vi "Manual CAN Send Cammand.vi"() -> ()   [LabVIEW 2015]
panel:
  in  "stop":bool
  out "number":u32[](array[numeric])
  out "appended array":string[](array[string])
  out "all rows":string[][](array[string])
  in  "CAN  Send Cammand":bool
  in  "Responce Cammand":string
  in  "Cammand Test":u16(ring) items=["Send req seed send key to test sample", "Send Diag command to sample", "Buzzer ON", "Buzzer OFF", "End Activation command to test sample", "Send req seed send key to master", "Send Diag command to master", "Send req seed send key to test sample", "Send Diag command to Test sample", "Dial Illumination ON for master", "Pointer Illumination ON for master", "LCD Illumination ON for master", "Dial Illumination ON for Test Sample", "Pointer Illumination ON for Test Sample", "LCD Illumination ON for Test Sample", "LCD All Seg ON to master", "LCD All Seg ON to test sample", "LCD All segment OFF to master", "LCD All segment OFF to test sample", "End Activation command to master", "End Activation command to test sample", "All telltale ON command to master", "All telltale ON command to test sample", "All telltlae OFF command to master", "All telltlae OFF command to test sample", "End Activation command for Master", "End Activation command for Test", "Move Speedo to 0 km/hr to master", "Move Speedo to 0 km/hr to Test sample", "Move speedo to 20 km/hr to master", "Move speedo to 20 km/hr to test sample", "Move speedo to 40 km/hr to master", "Move speedo to 40 km/hr to test sample", "Move speedo to 60 km/hr to master", "Move speedo to 60 km/hr to test sample", "Move Speedo to 80 km/hr to master", "Move Speedo to 80 km/hr to test sample", "Move speedo to 100 km/hr to master", "Move speedo to 100 km/hr to test sample", "Move Speedo to 120 to master", "Move Speedo to 120 to test sample", "Move speedo to 140 km/hr to master", "Move speedo to 140 km/hr to test sample", "Move speedo to 160 km/hr to master", "Move speedo to 160 km/hr to test sample", "Move Speedo to 180 to master", "Move Speedo to 180 to test sample", "End Activation for Testing Sample", "Send req seed send key to test sample", "Send Diag command to Test sample", "CLEAR DTC LID 95", "CLEAR DTC LID 96", "CLEAR DTC LID 97", "CLEAR DTC LID 98", "CLEAR DTC LID 99", "CLEAR DTC LID 9A", "CLEAR DTC LID 9B", "CLEAR DTC LID 9C", "CLEAR DTC LID 9D", "CLEAR DTC LID 9E", "CLEAR DTC LID 9F", "CLEAR DTC LID A0", "CLEAR DTC LID A1", "CLEAR DTC LID A2", "CLEAR DTC LID A3", "CLEAR DTC LID A4", "CLEAR DTC LID A5", "CLEAR DTC LID A6", "CLEAR DTC LID A7", "CLEAR DTC LID A8", "CLEAR DTC LID A9", "CLEAR DTC LID AA", "READ DTC LID 95", "Read Request", "End Activation command to Master sample", "End Activation command to test sample"]
  out "Cammand":string
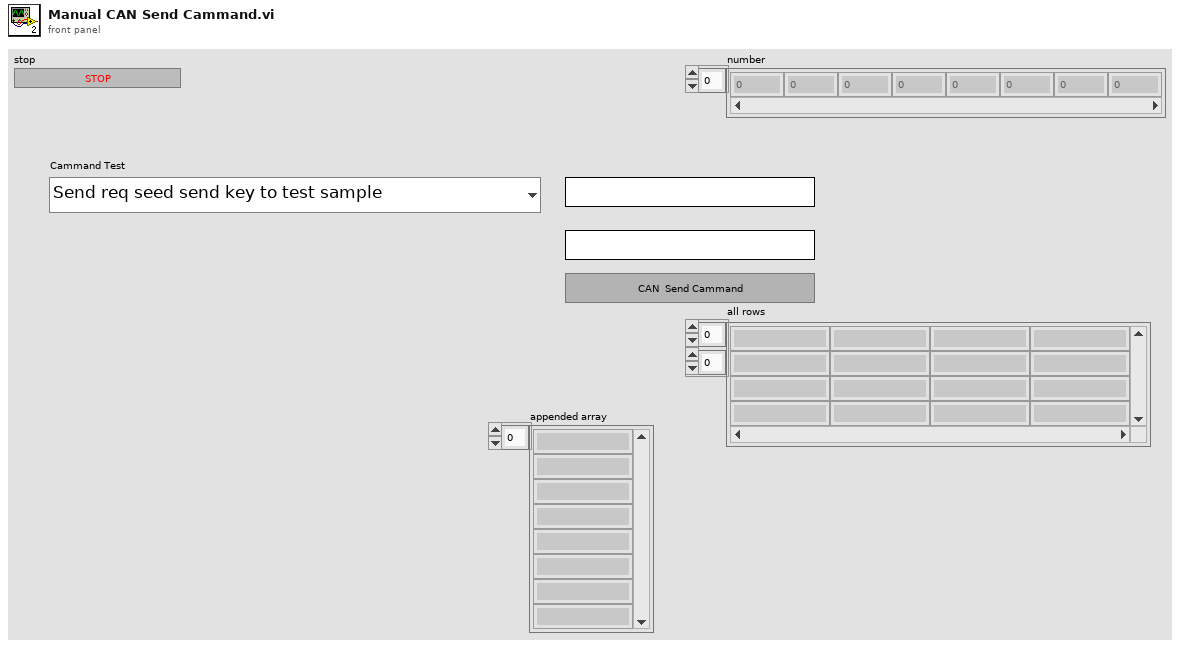
[diagram p1: front panel]
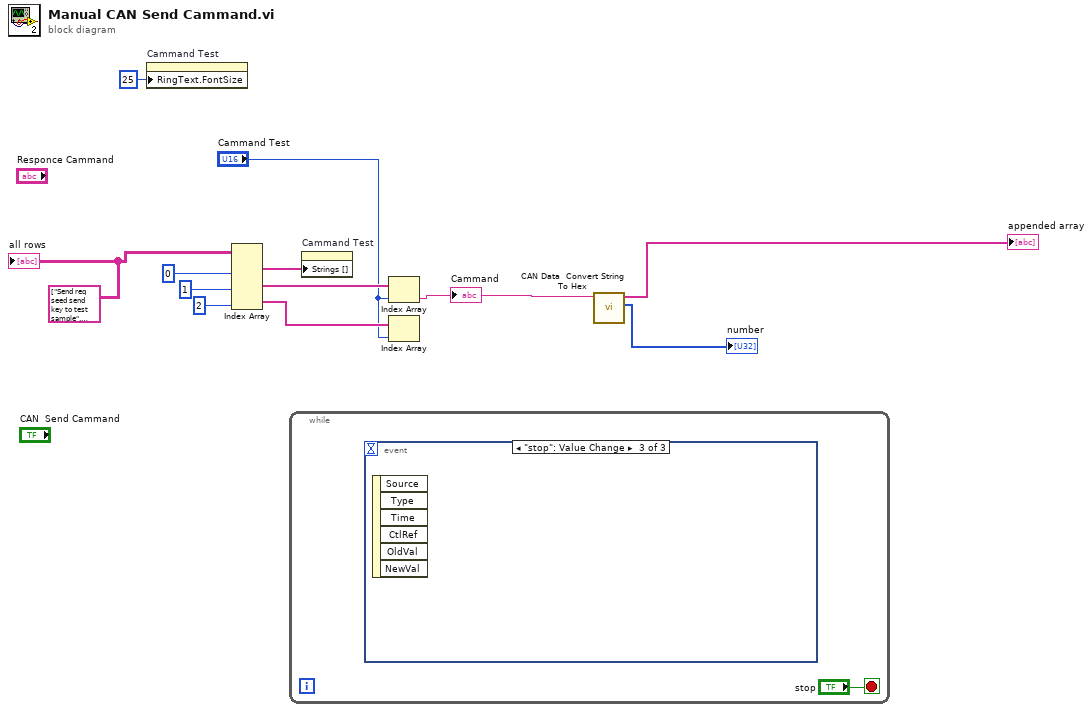
[diagram p0: block diagram]
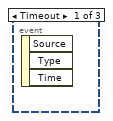
[diagram p2: hidden frame]
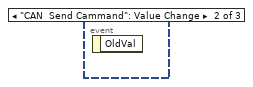
[diagram p3: hidden frame]
diagram:
  w1 = string[][] [["Send req seed send key to test sample", "0227FB0000000000", "0667FB", "0627FC", "0367FC34", "1", "0227FC", "0", "CAN0", "0", ""], ["Send Diag command to sample", "0210FA", "0250FA", "", "0", "0", "", "0", "CAN0", "0", ""], ["Buzzer ON", "0730130780800A00", "03701307", "", "", "0", "2", "0", "CAN0", "0", ""], ["Buzzer OFF", "0730130780800000", "03701307", "", "", "0", "", "0", "CAN0", "", ""], ["End Activation command to test sample", "0120", "0160", "", "", "0", "", "0", "CAN0", "0", ""], ["Send req seed send key to master", "0227FB0000000000", "0667FB", "0627FC", "0367FC34", "1", "24", "0", "CAN1", "0", ""], ["Send Diag command to master", "0210FA", "0250FA", "", "0", "0", "24", "0", "CAN1", "0", ""], ["Send req seed send key to test sample", "0227FB0000000000", "0667FB", "0627FC", "0367FC34", "1", "3", "0", "CAN0", "0", ""], ["Send Diag command to Test sample", "0210FA", "0250FA", "", "0", "0", "3", "0", "CAN0", "0", ""], ["Dial Illumination ON for master", "0631840100FFFF00", "027184", "", "", "0", "24", "0", "CAN1", "0", ""], ["Pointer Illumination ON for master", "0631840101FFFF00", "027184", "", "", "0", "24", "0", "CAN1", "0", ""], ["LCD Illumination ON for master", "0631840102FFFF00", "027160", "", "", "0", "24", "0", "CAN1", "0", ""], ["Dial Illumination ON for Test Sample", "0631840100FFFF00", "027184", "", "", "0", "4", "0", "CAN0", "0", ""], ["Pointer Illumination ON for Test Sample", "0631840101FFFF00", "027184", "", "", "0", "4", "0", "CAN0", "0", ""], ["LCD Illumination ON for Test Sample", "0631840102FFFF00", "027160", "", "", "0", "4", "0", "CAN0", "0", ""], ["LCD All Seg ON to master", "0431602100000000", "027160", "", "", "0", "24", "0", "CAN1", "0", ""], ["LCD All Seg ON to test sample", "0431602100000000", "027160", "", "", "0", "4", "0", "CAN0", "0", ""], ["LCD All segment OFF to master", "0431604100000000", "027160", "56", "0", "0", "24", "0", "CAN1", "0", ""], ["LCD All segment OFF to test sample", "0431604100000000", "027160", "56", "0", "0", "5", "0", "CAN0", "0", ""], ["End Activation command to master", "0120", "0160", "", "", "0", "24", "0", "CAN1", "0", ""], ["End Activation command to test sample", "0120", "0160", "", "", "0", "", "0", "CAN0", "0", ""], ["All telltale ON command to master", "0431342100", "027134", "", "", "0", "24", "1", "CAN1", "0", ""], ["All telltale ON command to test sample", "0431342100", "027134", "", "", "0", "6", "1", "CAN0", "0", ""], ["All telltlae OFF command to master", "0431344100", "027134", "", "", "0", "24", "1", "CAN1", "0", ""], ["All telltlae OFF command to test sample", "0431344100", "027134", "", "", "0", "7", "1", "CAN0", "0", ""], ["End Activation command for Master", "0120", "", "", "", "0", "24", "0", "CAN1", "0", ""], ["End Activation command for Test", "0120", "", "", "", "0", "8", "0", "CAN0", "0", ""], ["Move Speedo to 0 km/hr to master", "0000000000000000", "", "", "", "0", "24", "1", "CAN1", "788", ""], ["Move Speedo to 0 km/hr to Test sample", "0000000000000000", "", "", "", "0", "9", "1", "CAN0", "788", ""], ["Move speedo to 20 km/hr to master", "000A000000000000", "", "", "", "0", "24", "1", "CAN1", "788", ""], ["Move speedo to 20 km/hr to test sample", "000A000000000000", "", "", "", "0", "10", "1", "CAN0", "788", ""], ["Move speedo to 40 km/hr to master", "0014000000000000", "", "", "", "0", "24", "1", "CAN1", "788", ""], ["Move speedo to 40 km/hr to test sample", "0014000000000000", "", "", "", "0", "11", "1", "CAN0", "788", ""], ["Move speedo to 60 km/hr to master", "001E000000000000", "", "", "", "0", "24", "1", "CAN1", "788", ""], ["Move speedo to 60 km/hr to test sample", "001E000000000000", "", "", "", "0", "12", "1", "CAN0", "788", ""], ["Move Speedo to 80 km/hr to master", "0028000000000000", "", "", "", "0", "24", "1", "CAN1", "788", ""], ["Move Speedo to 80 km/hr to test sample", "0028000000000000", "", "", "", "0", "13", "1", "CAN0", "788", ""], ["Move speedo to 100 km/hr to master", "0032000000000000", "", "", "", "0", "24", "1", "CAN1", "788", ""], ["Move speedo to 100 km/hr to test sample", "0032000000000000", "", "", "", "0", "14", "1", "CAN0", "788", ""], ["Move Speedo to 120 to master", "003C000000000000", "", "", "", "0", "24", "1", "CAN1", "788", ""], ["Move Speedo to 120 to test sample", "003C000000000000", "", "", "", "0", "15", "1", "CAN0", "788", ""], ["Move speedo to 140 km/hr to master", "0046000000000000", "", "", "", "0", "24", "1", "CAN1", "788", ""], ["Move speedo to 140 km/hr to test sample", "0046000000000000", "", "", "", "0", "16", "1", "CAN0", "788", ""], ["Move speedo to 160 km/hr to master", "0050000000000000", "", "", "", "0", "24", "1", "CAN1", "788", ""], ["Move speedo to 160 km/hr to test sample", "0050000000000000", "", "", "", "0", "17", "1", "CAN0", "788", ""], ["Move Speedo to 180 to master", "005A000000000000", "", "", "", "0", "24", "1", "CAN1", "788", ""], ["Move Speedo to 180 to test sample", "005A000000000000", "", "", "", "0", "18", "1", "CAN0", "788", ""], ["End Activation for Testing Sample", "0120", "0160", "", "", "0", "", "0", "CAN0", "628", ""], ["Send req seed send key to test sample", "0227FB0000000000", "0667FB", "0627FC", "0367FC34", "1", "3", "0", "CAN0", "0", ""], ["Send Diag command to Test sample", "0210FA0000000000", "0250FA", "", "0", "0", "3", "0", "CAN0", "0", ""], ["CLEAR DTC LID 95", "0314FF000", "027161", "", "", "0", "22", "0", "CAN0", "0", ""], ["CLEAR DTC LID 96", "053161819600", "027161", "", "", "0", "", "0", "CAN0", "", ""], ["CLEAR DTC LID 97", "053161819700", "027161", "", "", "0", "", "0", "CAN0", "", ""], ["CLEAR DTC LID 98", "053161819800", "027161", "", "", "0", "", "0", "CAN0", "", ""], ["CLEAR DTC LID 99", "053161819900", "027161", "", "", "0", "", "0", "CAN0", "", ""], ["CLEAR DTC LID 9A", "053161819A00", "027161", "", "", "0", "", "0", "CAN0", "", ""], ["CLEAR DTC LID 9B", "053161819B00", "027161", "", "", "0", "", "0", "CAN0", "", ""], ["CLEAR DTC LID 9C", "053161819C00", "027161", "", "", "0", "", "0", "CAN0", "", ""], ["CLEAR DTC LID 9D", "053161819D00", "027161", "", "", "0", "", "0", "CAN0", "", ""], ["CLEAR DTC LID 9E", "053161819E00", "027161", "", "", "0", "", "0", "CAN0", "", ""], ["CLEAR DTC LID 9F", "053161819F00", "027161", "", "", "0", "", "0", "CAN0", "", ""], ["CLEAR DTC LID A0", "05316181A000", "027161", "", "", "0", "", "0", "CAN0", "", ""], ["CLEAR DTC LID A1", "05316181A100", "027161", "", "", "0", "", "0", "CAN0", "", ""], ["CLEAR DTC LID A2", "05316181A200", "027161", "", "", "0", "", "0", "CAN0", "", ""], ["CLEAR DTC LID A3", "05316181A300", "027161", "", "", "0", "", "0", "CAN0", "", ""], ["CLEAR DTC LID A4", "05316181A400", "027161", "", "", "0", "", "0", "CAN0", "", ""], ["CLEAR DTC LID A5", "05316181A500", "027161", "", "", "0", "", "0", "CAN0", "", ""], ["CLEAR DTC LID A6", "05316181A600", "027161", "", "", "0", "", "0", "CAN0", "", ""], ["CLEAR DTC LID A7", "05316181A700", "027161", "", "", "0", "", "0", "CAN0", "", ""], ["CLEAR DTC LID A8", "05316181A800", "027161", "", "", "0", "", "0", "CAN0", "", ""], ["CLEAR DTC LID A9", "05316181A900", "027161", "", "", "0", "", "0", "CAN0", "", ""], ["CLEAR DTC LID AA", "05316181AA00", "027161", "", "", "0", "", "0", "CAN0", "", ""], ["READ DTC LID 95", "0431610195000000", "02716100", "", "", "0", "", "0", "CAN0", "", ""], ["Read Request", "0233610000000000", "0373610000000000", "", "", "0", "", "0", "CAN0", "", ""], ["End Activation command to Master sample", "0120", "", "", "", "0", "24", "0", "CAN1", "628", ""], ["End Activation command to test sample", "0120", "", "", "", "1", "8", "0", "CAN0", "0", ""]] ("all rows")
  n1 = property on="Cammand Test" class="Ring (strict)"("RingText.FontSize"=u32 25 ("Ring Text.Font:Size")) -> ()  [unwired: 2 in, 2 out]
  n2 = Index Array(array=w1, index (col) #1=0 ("disabled index (col)"), index (col) #2=1 ("index (col)"), index (col) #3=2 ("index (col)")) -> (element #1=w12:string[], element #2=w8:string[], element #3=w7:string[])  [unwired: 3 in]
  n3 = while {
    stop <- "stop" stop-if-true
    n4 = event shown="[2] \"stop\": Value Change" {
      selector: _ -> [_ _ _]
      dyn-events: _ -> [_ _ _]
      timeout: _ -> [_ _ _]
      event Timeout {
        n5 = event-data() -> ()  [unwired: 1 in, 3 out]
      }
      event "CAN  Send Cammand": Value Change {
        n6 = event-data() -> ()  [unwired: 1 in, 1 out]
      }
      event "stop": Value Change {
        n7 = event-data() -> ()  [unwired: 1 in, 6 out]
      }
    }
  }
  n8 = property on="Cammand Test" class="Ring (strict)"("Strings []"=w12) -> ()  [unwired: 2 in, 2 out]
  n9 = Index Array(array=w8, index="Cammand Test") -> (element=w4:string)
  "Cammand" <- w4
  n10 = Index Array(array=w7, index="Cammand Test") -> ()  [unwired: 1 out]
  n11 = call "CAN Data  Convert String To Hex.vi"("String"=w4) -> ("number"=→"number":u32[], "appended array"=→"appended array":string[])  [unwired: 9 in]
  "all rows" <- w1
